vi "choose operation.vi"(1 "Enum":T1(ring), 2 "channel":i8) -> ()   [LabVIEW 2023]
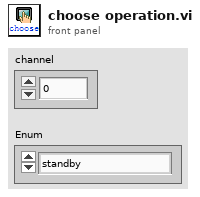
[diagram p1: front panel]
types:
  T1 = enum16{"standby", "pre-reaction", "reaction", "post-reaction", "analysis"}
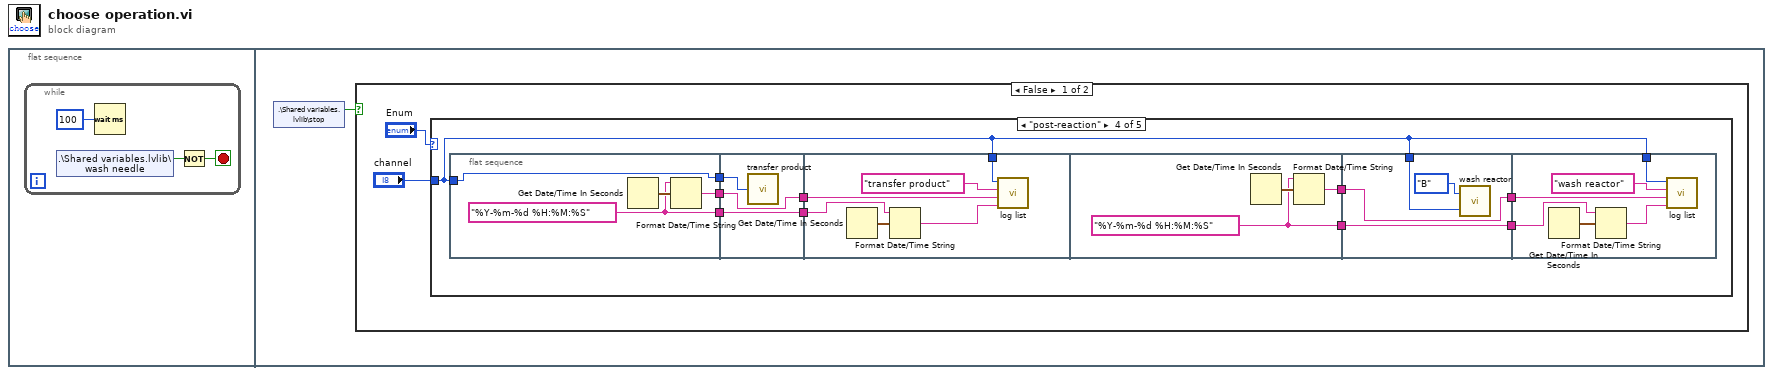
[diagram p0: block diagram]
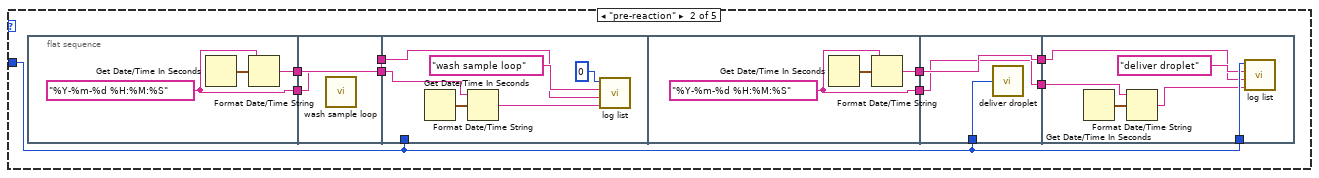
[diagram p3: hidden frame]
diagram:
  n1 = flat-sequence {
    frame #0 {
      n2 = while {
        stop <- w1 stop-if-true
        n3 = shared-variable ".\\Shared variables.lvlib\\wash needle"() -> (w2:bool)  [unwired: 1 in, 1 out]
        n4 = Wait (ms)(milliseconds to wait=u32 100) -> ()  [unwired: 1 out]
        n5 = Not(x=w2) -> (.not. x?=w1:bool)
      }
    }
    frame #1 {
      n6 = shared-variable ".\\Shared variables.lvlib\\stop"() -> (w4:bool)  [unwired: 1 in, 1 out]
      n7 = case shown="False" w4 {
        frame False {
          n8 = case shown="\"post-reaction\"" "Enum" {
            tunnel: "channel" -> [_ w7 _ w48 _]
            frame "standby", Default {
            }
            frame "pre-reaction" {
              n9 = flat-sequence {
                tunnel: [w17] -> w10
                tunnel: [w16] -> w8
                tunnel: [w20] -> w11
                tunnel: w10 -> [w20]
                tunnel: [w19] -> w9
                tunnel: w8 -> [w19]
                tunnel: w7 -> [_]
                tunnel: w11 -> [w23]
                tunnel: w9 -> [w21]
                tunnel: [w28] -> w14
                tunnel: [w27] -> w12
                tunnel: w7 -> [w32]
                tunnel: [w31] -> w15
                tunnel: w14 -> [w31]
                tunnel: [w30] -> w13
                tunnel: w12 -> [w30]
                tunnel: w7 -> [w38]
                tunnel: w15 -> [w36]
                tunnel: w13 -> [w33]
                frame #0 {
                  w16 = "%Y-%m-%d %H:%M:%S" ("time format string (%c)")
                  n10 = Get Date/Time In Seconds() -> (seconds since 1Jan1904=w18:timestamp)
                  n11 = Format Date/Time String(time format string (%c)=w16, seconds (now)=w18) -> (date/time string=w17:string)  [unwired: 1 in]
                }
                frame #1 {
                  n12 = call "wash sample loop.vi"() -> ()  [unwired: 12 in]
                }
                frame #2 {
                  n13 = Get Date/Time In Seconds() -> (seconds since 1Jan1904=w25:timestamp)
                  n14 = Format Date/Time String(time format string (%c)=w21, seconds (now)=w25) -> (date/time string=w26:string)  [unwired: 1 in]
                  n15 = call "log list.vi"("end"=w26, "start"=w23, "operaton"="wash sample loop" ("input string"), "worker"=i8 0) -> ()  [unwired: 7 in, 1 out]
                }
                frame #3 {
                  w27 = "%Y-%m-%d %H:%M:%S" ("time format string (%c)")
                  n16 = Get Date/Time In Seconds() -> (seconds since 1Jan1904=w29:timestamp)
                  n17 = Format Date/Time String(time format string (%c)=w27, seconds (now)=w29) -> (date/time string=w28:string)  [unwired: 1 in]
                }
                frame #4 {
                  n18 = call "deliver droplet.vi"("channel"=w32) -> ()  [unwired: 1 in]
                }
                frame #5 {
                  n19 = Get Date/Time In Seconds() -> (seconds since 1Jan1904=w35:timestamp)
                  n20 = Format Date/Time String(time format string (%c)=w33, seconds (now)=w35) -> (date/time string=w34:string)  [unwired: 1 in]
                  n21 = call "log list.vi"("end"=w34, "start"=w36, "operaton"="deliver droplet" ("input string"), "worker"=w38) -> ()  [unwired: 7 in, 1 out]
                }
              }
            }
            frame "reaction" {
            }
            frame "post-reaction" {
              n22 = flat-sequence {
                tunnel: w48 -> [w52]
                tunnel: [w52] -> w47
                tunnel: [w50] -> w46
                tunnel: [w49] -> w43
                tunnel: w47 -> [w55]
                tunnel: w46 -> [w54]
                tunnel: [w54] -> w45
                tunnel: [w53] -> w44
                tunnel: w43 -> [w53]
                tunnel: w48 -> [w58]
                tunnel: w45 -> [w57]
                tunnel: w44 -> [w56]
                tunnel: [w63] -> w41
                tunnel: [w62] -> w39
                tunnel: w48 -> [w66]
                tunnel: [w68] -> w42
                tunnel: w41 -> [w68]
                tunnel: [w67] -> w40
                tunnel: w39 -> [w67]
                tunnel: w48 -> [w71]
                tunnel: w42 -> [w70]
                tunnel: w40 -> [w69]
                frame #0 {
                  w49 = "%Y-%m-%d %H:%M:%S" ("time format string (%c)")
                  n23 = Get Date/Time In Seconds() -> (seconds since 1Jan1904=w51:timestamp)
                  n24 = Format Date/Time String(time format string (%c)=w49, seconds (now)=w51) -> (date/time string=w50:string)  [unwired: 1 in]
                }
                frame #1 {
                  n25 = call "transfer product.vi"("channel"=w55) -> ()  [unwired: 1 in]
                }
                frame #2 {
                  n26 = Get Date/Time In Seconds() -> (seconds since 1Jan1904=w61:timestamp)
                  n27 = Format Date/Time String(time format string (%c)=w56, seconds (now)=w61) -> (date/time string=w60:string)  [unwired: 1 in]
                  n28 = call "log list.vi"("end"=w60, "start"=w57, "operaton"="transfer product" ("input string"), "worker"=w58) -> ()  [unwired: 7 in, 1 out]
                }
                frame #3 {
                  w62 = "%Y-%m-%d %H:%M:%S" ("time format string (%c)")
                  n29 = Get Date/Time In Seconds() -> (seconds since 1Jan1904=w64:timestamp)
                  n30 = Format Date/Time String(time format string (%c)=w62, seconds (now)=w64) -> (date/time string=w63:string)  [unwired: 1 in]
                }
                frame #4 {
                  n31 = call "wash reactor.vi"("channel"=w66, "Switch to position (A/B)"=enum16{"A", "B"}."B") -> ()  [unwired: 1 in]
                }
                frame #5 {
                  n32 = Get Date/Time In Seconds() -> (seconds since 1Jan1904=w74:timestamp)
                  n33 = Format Date/Time String(time format string (%c)=w69, seconds (now)=w74) -> (date/time string=w73:string)  [unwired: 1 in]
                  n34 = call "log list.vi"("end"=w73, "start"=w70, "operaton"="wash reactor" ("input string"), "worker"=w71) -> ()  [unwired: 7 in, 1 out]
                }
              }
            }
            frame "analysis" {
            }
          }
        }
        frame True {
        }
      }
    }
  }
